vi "Periodically Flush Queue.vi"(8 "error in (no error)":errorcluster, 11 "Report Generator in":refnum<class "Report Generator.lvclass">) -> (0 "error out":errorcluster, 3 "Report Generator out":refnum<class "Report Generator.lvclass">)   [LabVIEW 2023, in "Report Generator.lvlib" / "Report Generator.lvclass"]
doc: "This routine flushes the report queue and passes the flushed data to the <b>Process Flushed Data</b> Utility"
uses:
  Library/Report Generator.lvclass
  Library/Report Generator.lvclass/Report Generator.ctl
  builds/Tools/QDMH.lvlibp/Library/QDMH.lvclass
  builds/Framework/Engine.lvlibp/Engine/Library/Engine.lvclass
  C:/Users/Public/Documents/Development/builds/Main/Docking.lvlibp/Prime Panel/PrimeDock.lvclass
  C:/Users/Public/Documents/Development/builds/Main/Docking.lvlibp/Docking/Docking.lvclass
  C:/Users/Public/Documents/Development/builds/Framework/Engine.lvlibp/Managed Actor/Library/Managed Actor.lvclass
  C:/Users/Public/Documents/Development/builds/Framework/Engine.lvlibp/Engine/Library/Engine.lvclass
  C:/Users/Public/Documents/Development/builds/Framework/Panel Manager.lvlibp/Library/Panel Actor.lvclass
  C:/Users/Public/Documents/Development/builds/Framework/Monitored Actor.lvlibp/Actor Monitor/Actor Monitor/Actor Monitor.lvclass
  C:/Users/Public/Documents/Development/builds/Framework/Actor Framework.lvlibp/1abvi3w/vi.lib/ActorFramework/Actor/Actor.lvclass
  C:/Users/Public/Documents/Development/Application/Prime Panels/Report Generator/Library/Report Generator.lvclass
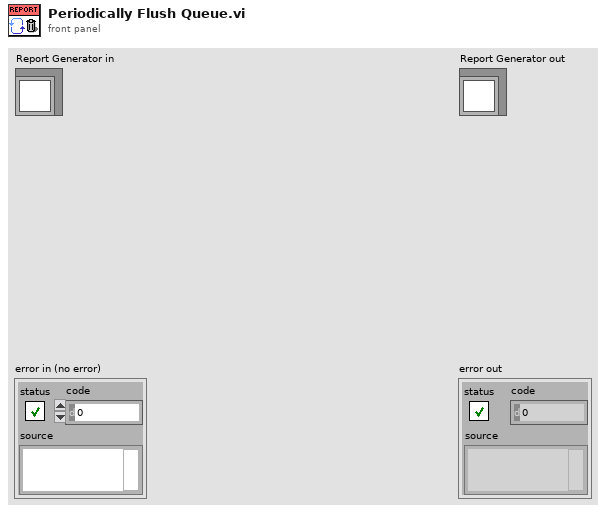
[diagram p1: front panel]
types:
  T1 = typedef "QDMH.lvlibp/QDMH.lvclass/Message.ctl" = cluster{"State":string, "Data":variant}
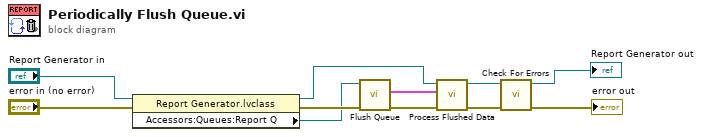
[diagram p0: block diagram]
diagram:
  n1 = property class="Report Generator.lvclass"(reference="Report Generator in", error in="error in (no error)") -> (reference out=w5:refnum<class "Report Generator.lvclass">, error out=w9:errorcluster, "Accessors:Queues:Report Q"=w8:refnum<class "QDMH.lvclass">)
  n2 = call "Flush Queue.vi"("error in (no error)"=w9, "QDMH in"=w8) -> ("error out"=w4:errorcluster, "Flushed Elements"=w1:T1[])  [unwired: 7 in, 1 out]
  n3 = call "Process Flushed Data.vi"("error in (no error)"=w4, "Flushed Elements"=w1, "Report Generator in"=w5) -> ("error out"=w3:errorcluster, "Report Generator out"=w2:refnum<class "Report Generator.lvclass">)  [unwired: 7 in]
  n4 = call "Check For Errors.vi"("error in"=w3, "Engine in"=w2) -> ("error out"=→"error out":errorcluster, "Engine out"=→"Report Generator out":refnum<class "Report Generator.lvclass">)  [unwired: 8 in]
